vi "Global.vi"() -> ()   [LabVIEW 2017, in "niFpgaDsp48e.xnode"]
uses:
  <vilib>/rvi/FXPMathLib/basic elements/DSP48E/XNode/niFpgaDsp48e.xnode
panel:
  in  "REPLACE MENU ID":string="DSP48E_MENU_REPLACE"
  out "dsp48e1 contracted warning banner":picture
  out "dsp48e1 contracted banner":picture
  in  "dsp48e1 banner":picture
  out "dsp48e contracted warning banner":picture
  out "dsp48e contracted banner":picture
  in  "terminal ID":string[](array[string])=["A_ID", "ACIN_ID", "B_ID", "BCIN_ID", "ACOUT_ID", "BCOUT_ID", "C_ID", "D_ID", "INMODE_ID", "P_ID", "PCIN_ID", "PCOUT_ID", "CARRYIN_ID", "CARRYOUT_ID", "CARRYCASCIN_ID", "CARRYCASCOUT_ID", "MULTSIGNIN_ID", "MULTSIGNOUT_ID", "ALUMODE_ID", "OPMODE_ID", "CARRYINSEL_ID", "PATTERNDETECT_ID", "PATTERNBDETECT_ID", "OVERFLOW_ID", "UNDERFLOW_ID", "CLEAR_ID", "RSTM_ID", "RSTALUMODE_ID", "RSTA_ID", "RSTB_ID", "RSTC_ID", "RSTD_ID", "RSTINMODE_ID", "RSTP_ID", "RSTCTRL_ID", "RSTALLCARRYIN_ID", "ENABLE_ID", "CEA1_ID", "CEA2_ID", "CEB1_ID", "CEB2_ID", "CEM_ID", "CEALUMODE_ID", "CEC_ID", "CEAD_ID", "CED_ID", "CEINMODE_ID", "CEP_ID", "CECTRL_ID", "CEMULTCARRYIN_ID", "CECARRYIN_ID"]
  in  "terminal name":string[](array[string])=["a", "acin", "b", "bcin", "acout", "bcout", "c", "d", "inmode", "p", "pcin", "pcout", "carryin", "carryout", "carrycascin", "carrycascout", "multsignin", "multsignout", "alumode", "opmode", "carryinsel", "patterndetect", "patternbdetect", "overflow", "underflow", "clear", "rstm", "rstalumode", "rsta", "rstb", "rstc", "rstd", "rstinmode", "rstp", "rstctrl", "rstallcarryin", "enable", "cea1", "cea2", "ceb1", "ceb2", "cem", "cealumode", "cec", "cead", "ced", "ceinmode", "cep", "cectrl", "cemultcarryin", "cecarryin"]
  in  "dsp48e banner":picture
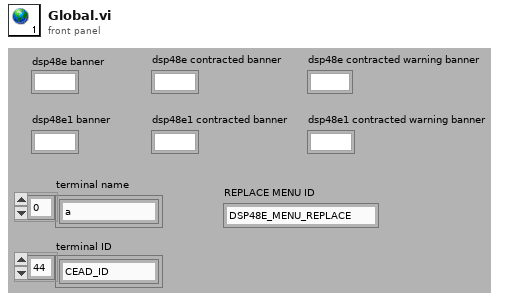
[diagram p1: front panel]
diagram:
